vi "encodercc.vi"() -> ()   [LabVIEW 2019]
uses:
  <vilib>/rvi/Emulation/niFpgaGetClockAttributes.vi
  <vilib>/rvi/Emulation/niFpgaSctlEmulationGetInTimedLoop.vi
  <vilib>/rvi/Emulation/niFpgaEmulationReportErrorSimple.vi
  <vilib>/rvi/eio/common/nirviEmuTemplateMethod_errors.vi
  <vilib>/rvi/Emulation/niFpgaCriticalErrorInLSC.vi
  <vilib>/eio/EIONode/EIONode.xnode
  <vilib>/rvi/Arithmetic/AddSubMult/XNode/nirviSatArithmetic.xnode
panel:
  in  "Position Reset":bool
  in  "Velocity Interval (uSec)":u32=1000
  out "Position (Counts)":i32
  out "Acceleration (Counts/Interval)":i32
  out "Velocity (Counts/Interval)":i32
  out "Loop time (position)":u32
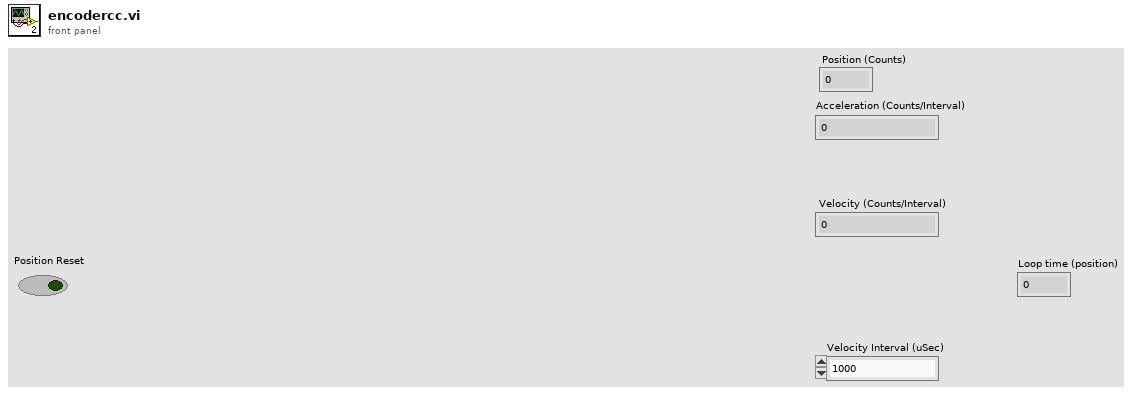
[diagram p1: front panel]
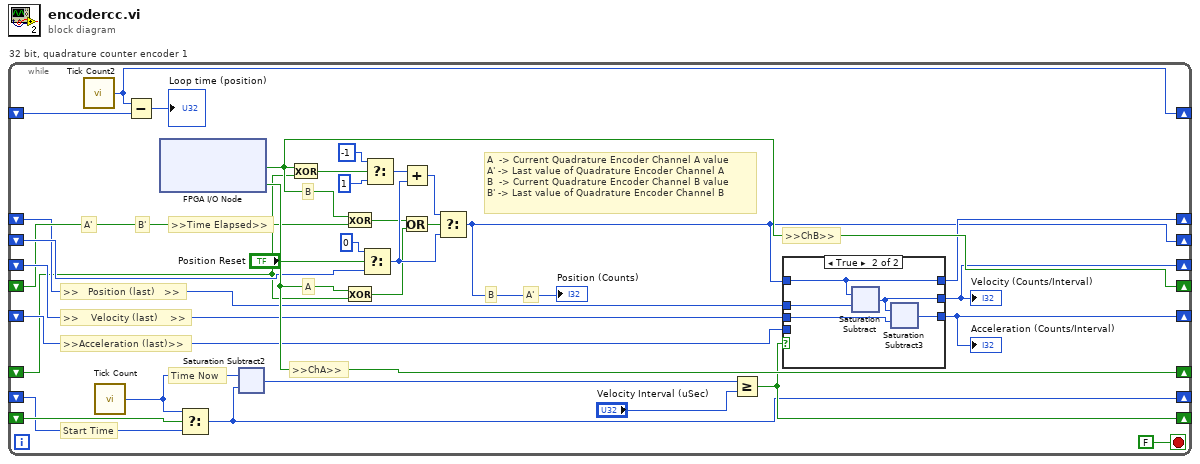
[diagram p0: block diagram]
diagram:
  n1 = while "32 bit, quadrature counter encoder 1" {
    shift-right: [w24] -> _
    shift-left: _ -> [w11]
    shift-right: [w7] -> _
    shift-left: _ -> [w21]
    shift-right: [w23] -> _
    shift-left: _ -> [w1]
    shift-right: [w17] -> _
    shift-left: _ -> [w20]
    shift-right: [w13] -> _
    shift-left: _ -> [w18]
    shift-right: [w8] -> _
    shift-left: _ -> [w6]
    shift-right: [w9] -> _
    shift-left: _ -> [w15]
    shift-right: [w10] -> _
    shift-left: _ -> [w12]
    shift-right: [w3] -> _
    shift-left: _ -> [w5]
    stop <- FALSE stop-if-true
    # "A  -> Current Quadrature Encoder Channel A value\nA' -> Last value of Quadrature Encoder Channel A\nB  -> Current Quadrature Encoder Channel B value\nB' -> Last value of Quadrature Encoder Channel B"
    # ">>Acceleration (last)>>"
    # "Start Time"
    # "A'"
    # "B"
    # "A'"
    # "A"
    # "B'"
    # "B"
    # ">>ChB>>"
    # ">>ChA>>"
    # ">>    Velocity (last)    >>"
    # ">>   Position (last)   >>"
    # "Time Now"
    # ">>Time Elapsed>>"
    n2 = call "Tick Count2"() -> ("Tick Count(Ticks)"=w3:u32)
    n3 = call "Tick Count"() -> ("Tick Count(uSec)"=w14:u32)
    n4 = Subtract(x=w3, y=w5) -> (x-y=→"Loop time (position)":u32)
    n5 = xnode "FPGA I/O Node"() -> ("RMC/DIO55"=w24:bool, "RMC/DIO54"=w23:bool)  [unwired: 2 in, 2 out]
    n6 = Select(t=w14, s=w20, f=w18) -> (s? t:f=w13:u32)
    n7 = xnode ("Saturation Subtract2")("x"=w14, "y"=w13) -> ("x-y"=w16:u32)
    n8 = Exclusive Or(1:w1, 2:w24) -> (0:w25:bool)
    n9 = Exclusive Or(1:w11, 2:w24) -> (0:w26:bool)
    n10 = Exclusive Or(1:w1, 2:w23) -> (0:w27:bool)
    n11 = Select(t=0 ("32 bit"), s="Position Reset", f=w21) -> (s? t:f=w32:i32)
    n12 = Select(t=-1 ("32 bit"), s=w25, f=1 ("32 bit")) -> (s? t:f=w30:i32)
    n13 = Add(x=w30, y=w32) -> (x+y=w34:i32)
    n14 = Or(x=w26, y=w27) -> (x .or. y?=w22:bool)
    n15 = Select(t=w34, s=w22, f=w32) -> (s? t:f=w7:i32)
    "Position (Counts)" <- w7
    n16 = Greater Or Equal?(x=w16, y="Velocity Interval (uSec)") -> (x >= y?=w17:bool)
    n17 = case shown="True" w17 {
      tunnel: w7 -> [_ w48]
      tunnel: w6 -> [w45 w52]
      tunnel: [w47 w51] -> w9
      tunnel: w15 -> [w47 w50]
      tunnel: [w46 w49] -> w10
      tunnel: w12 -> [w46 _]
      tunnel: [w45 w48] -> w8
      frame False {
      }
      frame True {
        n18 = xnode ("Saturation Subtract")("x"=w48, "y"=w52) -> ("x-y"=w51:i32)
        n19 = xnode ("Saturation Subtract3")("x"=w51, "y"=w50) -> ("x-y"=w49:i32)
      }
    }
    "Acceleration (Counts/Interval)" <- w10
    "Velocity (Counts/Interval)" <- w9
  }
